vi "Error Processor.vi"(8 "error in (no error)":errorcluster, 11 "Error Manager in":refnum<class "Error Manager.lvclass">) -> (0 "error out":errorcluster, 3 "Error Manager out":refnum<class "Error Manager.lvclass">)   [LabVIEW 2026, in "TALOS.lvlib" / "Error Manager.lvlib" / "Error Manager.lvclass"]
doc: "Use this VI to process all the error that are solvable inside this specific uService. Whatever is not possible to process, let it leave this VI and it will be processed by the Error Manager of the Distributed System."
uses:
  Error Manager.lvclass
  Father of all uServices/Father of all uServices/Father of all uServices.lvclass
  TALOS.lvlib
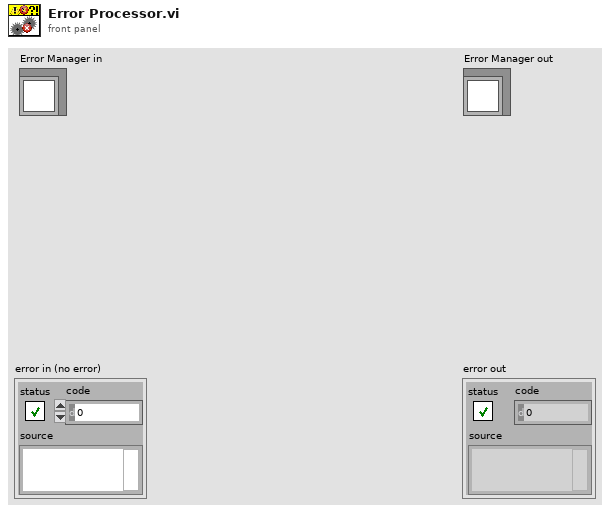
[diagram p1: front panel]
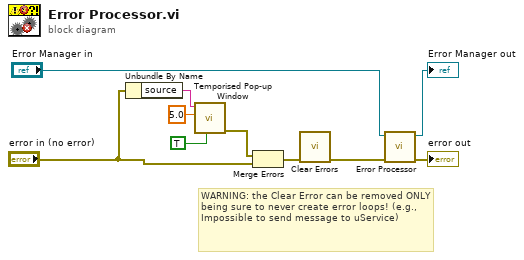
[diagram p0: block diagram]
diagram:
  # "WARNING: the Clear Error can be removed ONLY being sure to never create error loops! (e.g., Impossible to send message to uService)"
  n1 = Unbundle By Name("error in (no error)") -> ("source"=w4:string)
  n2 = call "Temporised Pop-up Window.vi"("error window"=TRUE, "Timeout"=5.0, "Text"=w4) -> ("error out"=w2:errorcluster)  [unwired: 8 in]
  n3 = Merge Errors(w2, "error in (no error)") -> (w3:errorcluster)
  n4 = call <vilib>:"Clear Errors.vi"("error in (no error)"=w3) -> ("error out"=w7:errorcluster)  [unwired: 5 in, 1 out]
  n5 = call-parent "Error Processor.vi"("error in (no error)"=w7, "Father of all uServices in"="Error Manager in") -> ("error out"=→"error out":errorcluster, "Father of all uServices out"=→"Error Manager out":refnum<class "Error Manager.lvclass">)  [unwired: 8 in]
